vi "Parse.vi"(8 "error in (no error)":errorcluster, 11 "Transform.Scale in":refnum<class "Transform.Scale.lvclass">) -> (0 "error out":errorcluster, 3 "Transform.Scale out":refnum<class "Transform.Scale.lvclass">)   [LabVIEW 2019, in "Transform.Scale.lvclass"]
uses:
  Transform.Scale.lvclass
  C:/Users/Albro/Documents/GitHub/AFM-Lithography/lvsrc/Classes/Parse/Transform/Transform.lvclass
  <vilib>/Utility/error.llb/whitespace.ctl
  Transform/Transform.lvclass/Transform.ctl
  Transform/Transform.lvclass
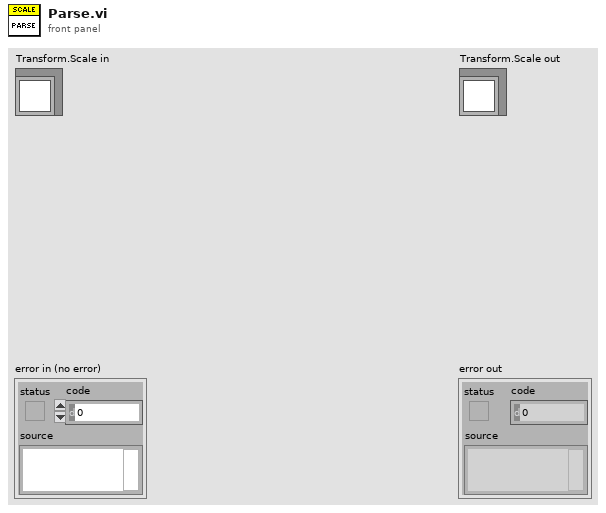
[diagram p1: front panel]
types:
  T1 = typedef "whitespace.ctl" = u16
  T2 = typedef "NI_Matrix.lvlib/RealMatrix.ctl" = dbl[][]
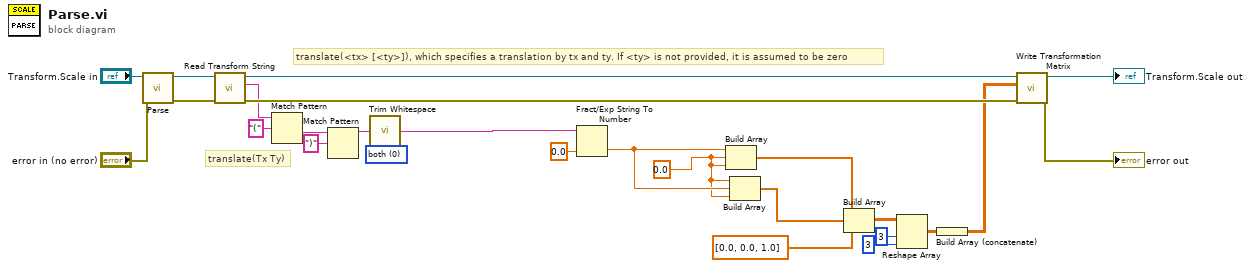
[diagram p0: block diagram]
diagram:
  w6 = 0.0 ("element")
  w16 = T1 0 items=["both", "start of string", "end of string"] ("location (both)")
  # "translate(<tx> [<ty>]), which specifies a translation by tx and ty. If <ty> is not provided, it is assumed to be zero"
  # "translate(Tx Ty)"
  n1 = call-parent "Parse.vi"("error in (no error)"="error in (no error)", "Transform in"="Transform.Scale in") -> ("error out"=w2:errorcluster, "Transform out"=w4:refnum<class "Transform.Scale.lvclass">)  [unwired: 8 in]
  n2 = call "Read Transform String.vi"("error in (no error)"=w2, "Transform in"=w4) -> ("error out"=w23:errorcluster, "Transform String"=w10:string, "Transform out"=w24:refnum<class "Transform.Scale.lvclass">)  [unwired: 7 in]
  n3 = Match Pattern(string=w10, regular expression="(") -> (after substring=w15:string)  [unwired: 1 in, 3 out]
  n4 = Match Pattern(string=w15, regular expression=")") -> (before substring=w20:string)  [unwired: 1 in, 3 out]
  n5 = call <vilib>:"Trim Whitespace.vi"("string"=w20, "location (both)"=w16) -> ("trimmed string"=w8:string)
  n6 = Fract/Exp String To Number(string=w8, default (0 dbl)=0.0 ("default (0 DBL)")) -> (number=w7:dbl)  [unwired: 2 in, 1 out]
  n7 = Build Array(w7, w6, w6) -> (w11:dbl[])
  n8 = Build Array(w6, w7, w6) -> (w5:dbl[])
  n9 = Build Array(w11, w5, dbl[] [0.0, 0.0, 1.0] ("element")) -> (w13:dbl[][])
  n10 = Reshape Array(w13, 3 ("dimension size"), 3 ("dimension size")) -> (w17:dbl[][])
  n11 = Build Array (concatenate)(w17) -> (w9:T2)
  n12 = call "Write Transformation Matrix.vi"("error in (no error)"=w23, "Real Matrix"=w9, "Transform in"=w24) -> ("error out"=→"error out":errorcluster, "Transform out"=→"Transform.Scale out":refnum<class "Transform.Scale.lvclass">)  [unwired: 7 in]
